vi "GetBit(U16).vi"() -> ()   [LabVIEW 2012]
panel:
  out "Bit":bool
  out "Bit(0or1)":i16
  in  "Bit(0-15)":u8
  in  "Input(U8)":u16 format="%.0x"
  out "error out":errorcluster caption="错误输出"
  in  "error in (no error)":errorcluster caption="错误输入（无错误）"
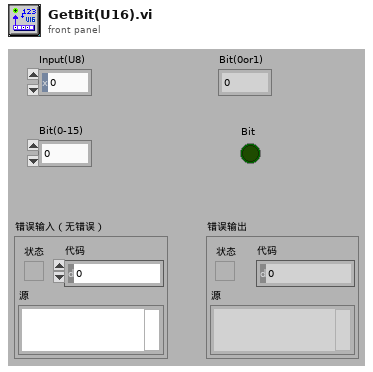
[diagram p1: front panel]
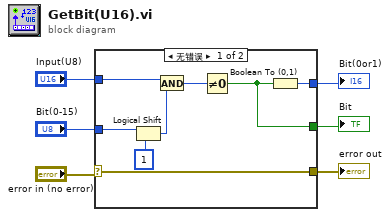
[diagram p0: block diagram]
diagram:
  n1 = case shown="无错误" "error in (no error)" {
    selector: "error in (no error)" -> [w14 w15]
    tunnel: [w14 w15] -> w5
    tunnel: "Bit(0-15)" -> [w12 _]
    tunnel: "Input(U8)" -> [w11 _]
    tunnel: [w8 _] -> w2
    tunnel: [w7 _] -> w1
    frame No Error {
      n2 = Logical Shift(y=w12, x=u16 1) -> (x << y=w10:u16)
      n3 = And(x=w11, y=w10) -> (x .and. y?=w9:u16)
      n4 = Not Equal To 0?(x=w9) -> (x != 0?=w8:bool)
      n5 = Boolean To (0,1)(Boolean=w8) -> (0, 1=w7:i16)
    }
    frame Error {
    }
  }
  "error out" <- w5
  "Bit" <- w2
  "Bit(0or1)" <- w1
